vi "Set Parent.vi"(8 "error in (no error)":errorcluster, 10 "Parent":refnum<data-value>, 11 "NodeRef In":refnum<data-value>) -> (0 "error out":errorcluster, 3 "NodeRef":refnum<data-value>)   [LabVIEW 2020, in "PicoG-ParserLexer.lvlib" / "Node.lvclass"]
doc: "Sets this node's parent if not already set. If this node already has a parent then RemoveChild must be called on the parent with this node first.\n\n<b>Error Codes:</b>\n<b>1556</b>: Node not instantiated with Ctor first, reference invalid.\n<b>14</b>: Parent is already assigned. Call RemoveChild on parent first."
uses:
  Node.lvclass
  <vilib>/ErrorRing/Error Ring.xnode
  <vilib>/Utility/error.llb/Error Cluster From Error Code.vi
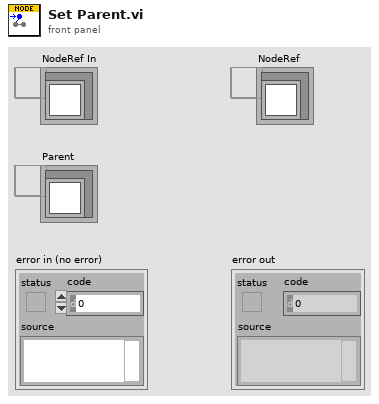
[diagram p1: front panel]
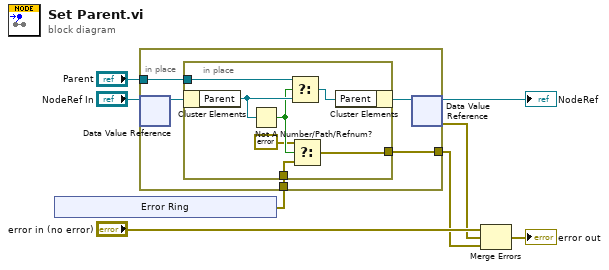
[diagram p0: block diagram]
diagram:
  n1 = xnode "Error Ring"() -> ("error out"=w4:errorcluster)
  n2 = in-place {
    in-place-border: "Parent" -> [w12]
    in-place-border: w4 -> [w10]
    in-place-border: [w9] -> w2
    n3 = in-place-dvr #1("NodeRef In") -> (w13:refnum<class "Node.lvclass">)  [unwired: 1 out]
    n4 = in-place {
      in-place-border: w12 -> [w19]
      in-place-border: w10 -> [w16]
      in-place-border: [w14] -> w9
      n5 = in-place-cluster #2(w13) -> ("Parent"=w20:refnum<data-value>)
      n6 = Not A Number/Path/Refnum?(number/path/refnum=w20) -> (NaN/Path/Refnum?=w17:bool)
      n7 = Select(t=w19, s=w17, f=w20) -> (s? t:f=w18:refnum<data-value>)
      n8 = Select(t=errorcluster {"status"=FALSE, "code"=0, "source"=""}, s=w17, f=w16) -> (s? t:f=w14:errorcluster)
      n9 = in-place-cluster #2("Parent"=w18) -> (w11:refnum<class "Node.lvclass">)
    }
    n10 = in-place-dvr #1(w11) -> (→"NodeRef":refnum<data-value>, w1:errorcluster)
  }
  n11 = Merge Errors("error in (no error)", w1, w2) -> (→"error out":errorcluster)
